vi "点阵图标定.vi"() -> ()   [LabVIEW 2018]
uses:
  <vilib>/vision/NI_Vision_Development_Module.lvlib
panel:
  out "ROI Descriptor":T1 {"Contours"."Type" items=["No Selection", "Point", "Line", "Rectangle", "Oval", "Polygon", "Freehand Region", "Annulus", "Unused2", "Unused3", "Broken Line", "Freehand Line", "Rotated Rectangle"]}
  in  "刷新按钮":bool
  in  "停止按钮":bool
  in  "确定按钮":bool
  in  "标定系数设置":cluster{"X轴方向间距":sgl, "Y轴方向间距":sgl, "单位选择":u16} {"单位选择" items=["Undefined", "Angstrom", "Micrometer", "Millimeter", "Centimeter", "Meter", "Kilometer", "Microinch", "Inch", "Feet", "Nautical miles", "Standardmiles", "Steps"]}
  out "二值化点阵图":T2(plugin-control)
  out "点阵图":T2(plugin-control)
  # "点阵图标定"
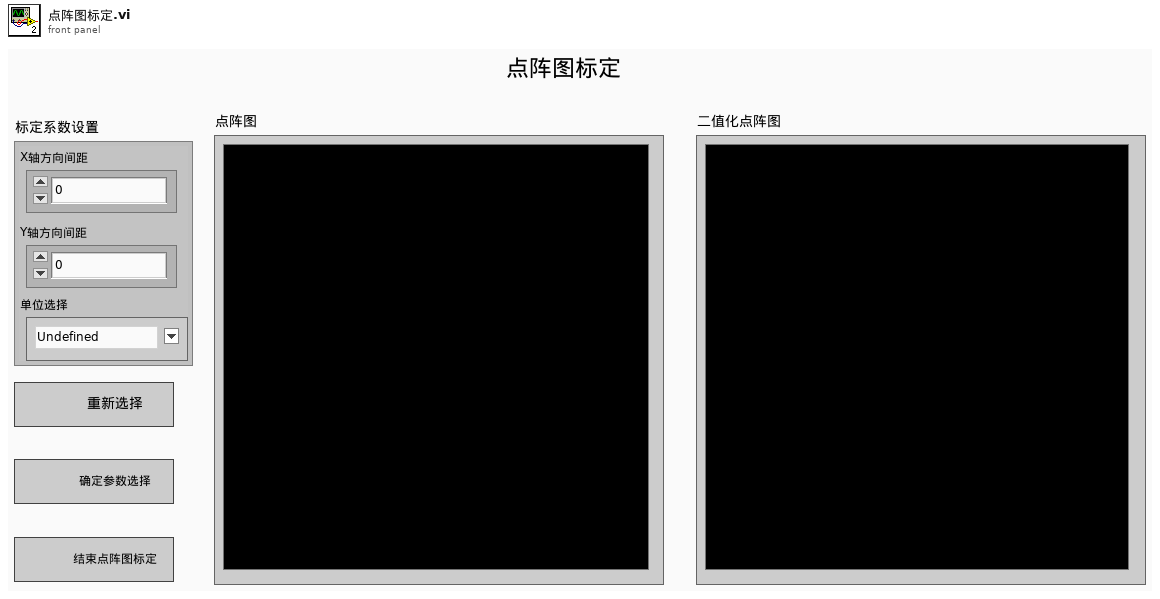
[diagram p1: front panel]
types:
  T1 = typedef "ROI Descriptor" = cluster{"Global Rectangle":i32[], "Contours":cluster{"ID":enum32{"External", "Internal"}, "Type":u32, "Coordinates":i32[]}[]}
  T2 = typedef "IMAQ Image.ctl" = refnum<image>
  T3 = enum8{"Enabled", "Disabled", "Disabled and Grayed Out"}
  T4 = enum32{"Invalid", "Standard", "Closed", "Hidden", "Minimized", "Maximized"}
  T5 = typedef "Image Type" = u32
  T6 = typedef "IMAQ Rectangle" = cluster{"Left":i32, "Top":i32, "Right":i32, "Bottom":i32, "Rotation":dbl}
  T7 = typedef "Calibration Reference Points.ctl" = cluster{"Pixel Coordinates":cluster{"X":dbl, "Y":dbl}[], "Real World Coordinates":cluster{"X":dbl, "Y":dbl}[], "Unit":T8, "Image Size":cluster{"X":u32, "Y":u32}}
  T8 = typedef "Image Unit" = enum32{"Undefined", "Angström", "Micrometer", "Millimeter", "Centimeter", "Meter", "Kilometer", "Microinch", "Inch", "Feet", "Nautical miles", "Standard miles", "Steps"}
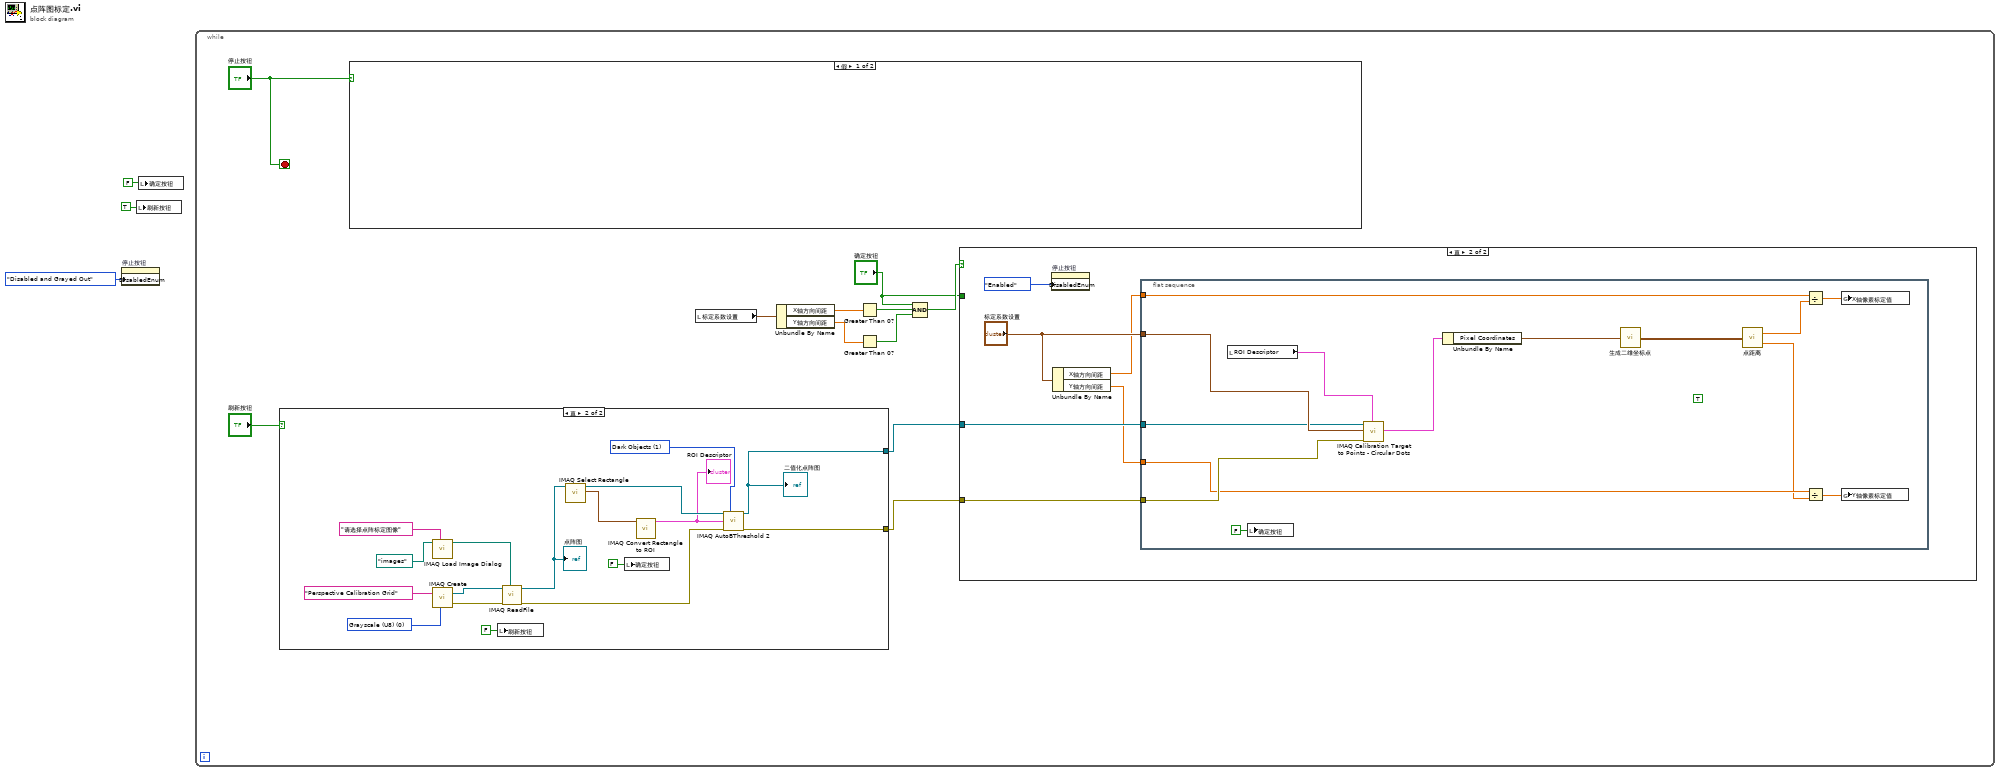
[diagram p0: block diagram]
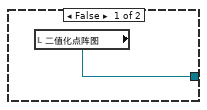
[diagram p2: hidden frame]
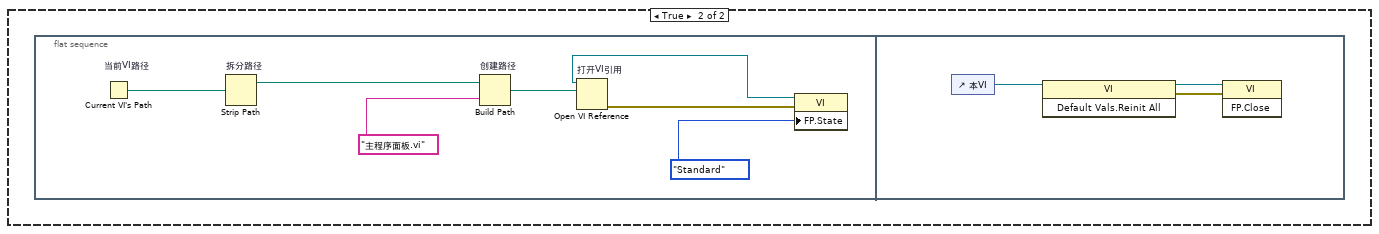
[diagram p3: hidden frame]
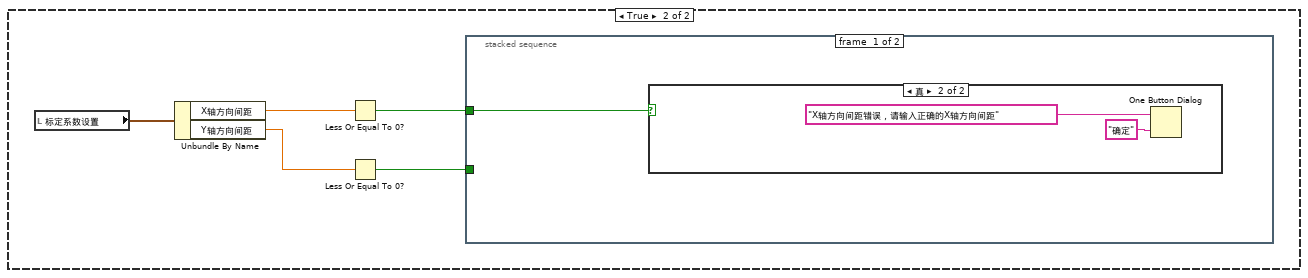
[diagram p5: hidden frame]
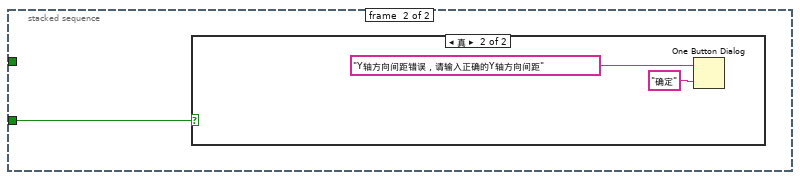
[diagram p7: hidden frame]
diagram:
  n1 = property on="停止按钮" class="Bool"("DisabledEnum"=T3."Disabled and Grayed Out" ("禁用")) -> ()  [unwired: 2 in, 2 out]
  n2 = local write "刷新按钮"(TRUE ("刷新按钮")) -> ()
  n3 = local write "确定按钮"(FALSE ("确定按钮")) -> ()
  n4 = while {
    stop <- "停止按钮" stop-if-true
    n5 = case shown="真" "刷新按钮" {
      tunnel: [w15 w21] -> w13
      tunnel: [_ w23] -> w12
      frame False {
        n6 = local read "二值化点阵图"() -> (w15:T2)
      }
      frame True {
        w32 = u32 1 items=["Bright Objects", "Dark Objects"] ("Look For (Bright Objects)")
        w30 = T5 0 items=["Grayscale (U8)", "Grayscale (I16)", "Grayscale (SGL)", "Complex (CSG)", "RGB (U32)", "HSL (U32)", "RGB (U64)", "Grayscale (U16)"] ("Image Type")
        n7 = call "IMAQ Load Image Dialog"("Prompt"="请选择点阵标定图像" ("prompt"), "Start Path"=path "images") -> ("Path"=w28:path)  [unwired: 7 in, 2 out]
        n8 = call "IMAQ Create"("Image Name"="Perspective Calibration Grid", "Image Type"=w30) -> ("New Image"=w25:T2, "error out"=w26:errorcluster)  [unwired: 2 in, 1 out]
        n9 = local write "刷新按钮"(FALSE ("刷新按钮")) -> ()
        n10 = call "IMAQ ReadFile"("File Path"=w28, "error in (no error)"=w26, "Image"=w25) -> ("error out"=w31:errorcluster, "Image Out"=w19:T2)  [unwired: 2 in, 5 out]
        "点阵图" <- w19
        n11 = call "IMAQ Select Rectangle"("Image In"=w19) -> ("Rectangle"=w17:T6, "Image Out (duplicate)"=w18:T2)  [unwired: 7 in, 2 out]
        n12 = local write "确定按钮"(FALSE ("刷新按钮")) -> ()
        n13 = call "IMAQ Convert Rectangle to ROI"("Rectangle"=w17) -> ("ROI Descriptor"=w16:T1)  [unwired: 8 in, 1 out]
        "ROI Descriptor" <- w16
        n14 = call "IMAQ AutoBThreshold 2"("Image Src"=w18, "Look For (Bright Objects)"=w32, "ROI Descriptor"=w16, "error in (no error)"=w31) -> ("Image Dst Out"=w21:T2, "error out"=w23:errorcluster)  [unwired: 9 in, 1 out]
        "二值化点阵图" <- w21
      }
    }
    n15 = case shown="假" "停止按钮" {
      frame False {
      }
      frame True {
        n16 = flat-sequence {
          frame #0 {
            n17 = Current VI's Path "当前VI路径"() -> (path=w37:path)
            n18 = Strip Path "拆分路径"(path=w37) -> (stripped path=w39:path)  [unwired: 1 out]
            n19 = Build Path "创建路径"(base path=w39, name or relative path="主程序面板.vi" ("名称或相对路径")) -> (appended path=w38:path)
            n20 = Open VI Reference "打开VI引用"(vi path=w38) -> (vi reference=w36:refnum<vi>, error out=w35:errorcluster)  [unwired: 5 in]
            n21 = property class="VI"(reference=w36, error in=w35, "FP.State"=T4."Standard" ("前面板窗口:状态")) -> ()  [unwired: 2 out]
          }
          frame #1 {
            n22 = control-ref of="本VI"() -> (w40:refnum<vi>)
            n23 = invoke class="VI" method="Default Vals.Reinit All"(reference=w40) -> (reference out=w41:refnum<vi>, error out=w42:errorcluster)  [unwired: 2 in, 1 out]
            n24 = invoke class="VI" method="FP.Close"(reference=w41, error in=w42) -> ()  [unwired: 1 in, 3 out]
          }
        }
      }
    }
    n25 = local read "标定系数设置"() -> (w10:cluster{"X轴方向间距":sgl, "Y轴方向间距":sgl, "单位选择":u16})
    n26 = Unbundle By Name(w10) -> ("X轴方向间距"=w9:sgl, "Y轴方向间距"=w8:sgl)
    n27 = Greater Than 0?(x=w9) -> (x > 0?=w6:bool)
    n28 = Greater Than 0?(x=w8) -> (x > 0?=w5:bool)
    n29 = Compound Arithmetic op=AND("确定按钮", w6, w5) -> (w7:bool)
    n30 = case shown="真" w7 {
      tunnel: w13 -> [_ w60]
      tunnel: w12 -> [_ w59]
      tunnel: "确定按钮" -> [w43 _]
      frame False {
        n31 = case shown="假" w43 {
          frame False {
          }
          frame True {
            n32 = local read "标定系数设置"() -> (w48:cluster{"X轴方向间距":sgl, "Y轴方向间距":sgl, "单位选择":u16})
            n33 = Unbundle By Name(w48) -> ("X轴方向间距"=w47:sgl, "Y轴方向间距"=w45:sgl)
            n34 = Less Or Equal To 0?(x=w47) -> (x <= 0?=w46:bool)
            n35 = Less Or Equal To 0?(x=w45) -> (x <= 0?=w44:bool)
            n36 = stacked-sequence {
              tunnel: w46 -> [w49 _]
              tunnel: w44 -> [_ w52]
              frame #0 {
                n37 = case shown="真" w49 {
                  frame False {
                  }
                  frame True {
                    n38 = One Button Dialog(message="X轴方向间距错误，请输入正确的X轴方向间距" ("消息"), button name ("OK")="确定" ("按钮名称（“确定”）")) -> ()  [unwired: 1 out]
                  }
                }
              }
              frame #1 {
                n39 = case shown="真" w52 {
                  frame False {
                  }
                  frame True {
                    n40 = One Button Dialog(message="Y轴方向间距错误，请输入正确的Y轴方向间距" ("消息"), button name ("OK")="确定" ("按钮名称（“确定”）")) -> ()  [unwired: 1 out]
                  }
                }
              }
            }
          }
        }
      }
      frame True {
        n41 = property on="停止按钮" class="Bool"("DisabledEnum"=T3."Enabled" ("禁用")) -> ()  [unwired: 2 in, 2 out]
        n42 = Unbundle By Name("标定系数设置") -> ("X轴方向间距"=w56:sgl, "Y轴方向间距"=w55:sgl)
        n43 = flat-sequence {
          tunnel: "标定系数设置" -> [w74]
          tunnel: w60 -> [w72]
          tunnel: w59 -> [w71]
          tunnel: w56 -> [w65]
          tunnel: w55 -> [w64]
          frame #0 {
            (unwired) TRUE ("Return Error Information (False)")
            n44 = local read "ROI Descriptor"() -> (w70:T1)
            n45 = local write "确定按钮"(FALSE ("确定按钮")) -> ()
            n46 = call "IMAQ Calibration Target to Points - Circular Dots"("ROI Descriptor"=w70, "error in (no error)"=w71, "Grid Descriptor"=w74, "Target Image"=w72) -> ("Reference Points"=w69:T7)  [unwired: 1 in, 6 out]
            n47 = Unbundle By Name(w69) -> ("Pixel Coordinates"=w68:cluster{"X":dbl, "Y":dbl}[])
            n48 = call "生成二维坐标点.vi"("输入无序一维坐标点"=w68) -> ("输出有序二维坐标点"=w67:cluster{"X":sgl, "Y":sgl}[][])
            n49 = call "点距离.vi"("二维点阵"=w67) -> ("X间距"=w66:sgl, "Y间距"=w63:sgl)
            n50 = Divide(x=w65, y=w66) -> (x/y=w62:sgl)
            n51 = Divide(x=w64, y=w63) -> (x/y=w61:sgl)
            n52 = global write "全局变量.vi" "X轴像素标定值"(w62) -> ()
            n53 = global write "全局变量.vi" "Y轴像素标定值"(w61) -> ()
          }
        }
      }
    }
  }
